vi "Split Raw Data.vi"(8 "error in (no error)":errorcluster, 9 "Accessors:RGB Gains":T1, 10 "Matrix":u32[][](array[colorbox])) -> (0 "error out":errorcluster, 3 "Array":u8[](array[numeric]))   [LabVIEW 2019, in "Display.lvclass"]
uses:
  Display.lvclass
  Public/Controls/RGB Gains.ctl
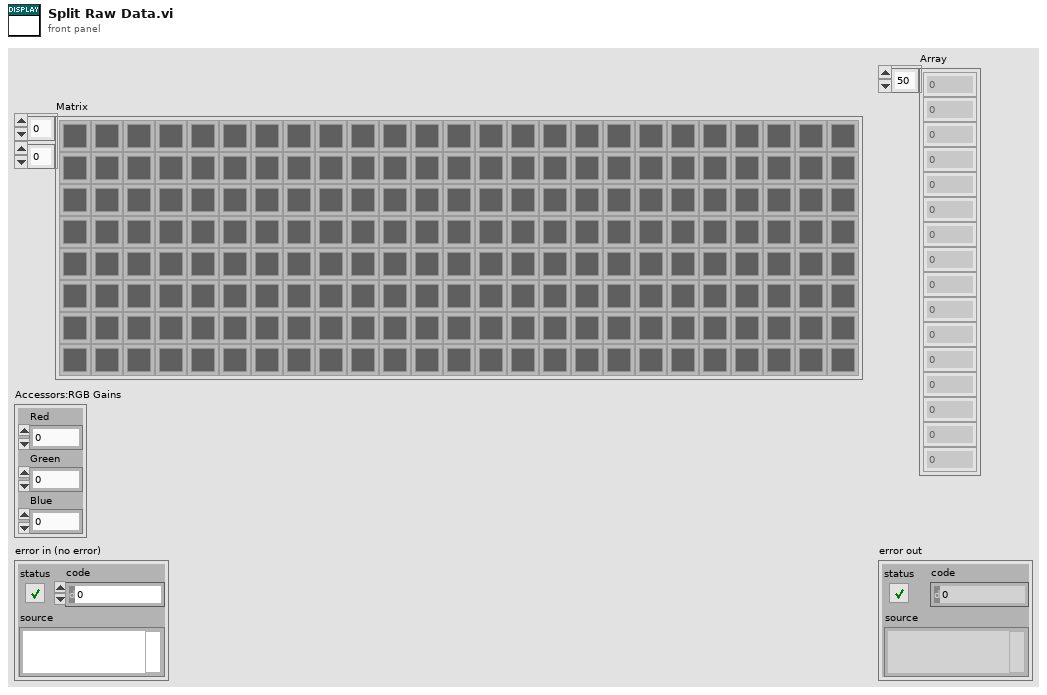
[diagram p1: front panel]
types:
  T1 = typedef "Display.lvclass/RGB Gains.ctl" = cluster{"Red":sgl, "Green":sgl, "Blue":sgl}
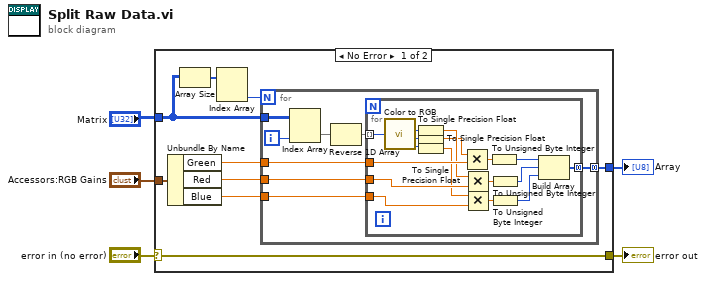
[diagram p0: block diagram]
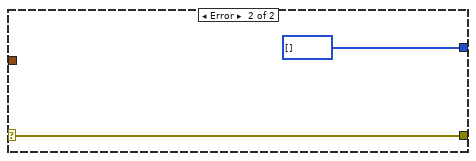
[diagram p2: hidden frame]
diagram:
  n1 = case shown="No Error" "error in (no error)" {
    selector: "error in (no error)" -> [w12 w41]
    tunnel: [w14 u8[] []] -> w5
    tunnel: "Accessors:RGB Gains" -> [w13 _]
    tunnel: "Matrix" -> [w7 _]
    tunnel: [w12 w41] -> w1
    frame No Error {
      n2 = Unbundle By Name(w13) -> ("Green"=w11:sgl, "Red"=w10:sgl, "Blue"=w9:sgl)
      n3 = Array Size(array=w7) -> (size(s)=w8:i32[])
      n4 = Index Array(array=w8) -> (element #2=w6:i32)  [unwired: 2 in, 1 out]
      n5 = for {
        N: w6 -> [_]
        tunnel: w11 -> [w22]
        tunnel: w10 -> [w21]
        tunnel: w9 -> [w20]
        tunnel: [w19] -> w14 mode=concatenating
        tunnel: w7 -> [w18]
        i -> [w15]
        n6 = Index Array(array=w18, index (col)=w15) -> (element=w17:u32[])  [unwired: 1 in]
        n7 = Reverse 1D Array(array=w17) -> (reversed array=w16:u32[])
        n8 = for {
          tunnel: w16 -> [w39] mode=indexing
          tunnel: [w38] -> w19 mode=concatenating
          tunnel: w22 -> [w32]
          tunnel: w21 -> [w31]
          tunnel: w20 -> [w30]
          n9 = call <vilib>:"Color to RGB.vi"("Color"=w39) -> ("R"=w29:u8, "G"=w27:u8, "B"=w25:u8)  [unwired: 1 out]
          n10 = To Single Precision Float(number=w29) -> (single precision float=w28:sgl)
          n11 = To Single Precision Float(number=w27) -> (single precision float=w26:sgl)
          n12 = To Single Precision Float(number=w25) -> (single precision float=w24:sgl)
          n13 = Multiply(x=w26, y=w32) -> (x*y=w37:sgl)
          n14 = Multiply(x=w28, y=w31) -> (x*y=w35:sgl)
          n15 = Multiply(x=w24, y=w30) -> (x*y=w23:sgl)
          n16 = To Unsigned Byte Integer(number=w37) -> (unsigned 8bit integer=w36:u8)
          n17 = To Unsigned Byte Integer(number=w35) -> (unsigned 8bit integer=w34:u8)
          n18 = To Unsigned Byte Integer(number=w23) -> (unsigned 8bit integer=w33:u8)
          n19 = Build Array(w36, w34, w33) -> (w38:u8[])
        }
      }
    }
    frame Error {
    }
  }
  "Array" <- w5
  "error out" <- w1
